vi "prep state ui channel.vi"(7 "instance id":string, 8 "error in":errorcluster, 9 "channel":refnum<class "TBM channel.lvclass">, 10 "ring":refnum<vi>, 11 "engine configuration in":refnum<class "engine configuration.lvclass">) -> (0 "error out":errorcluster, 3 "engine configuration out":refnum<class "engine configuration.lvclass">)   [LabVIEW 2013, in "user tag bus module editor node.lvclass"]
uses:
  user tag bus module editor node.lvclass
  <vilib>/NI/Tag Bus Module Framework/channel/TBM channel.lvclass
  <vilib>/NI/Module Execution Interface/Engine Configuration/engine configuration.lvclass
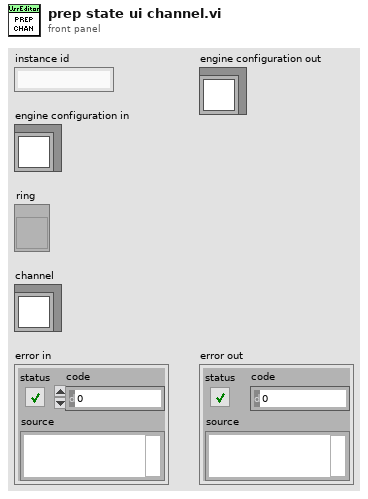
[diagram p1: front panel]
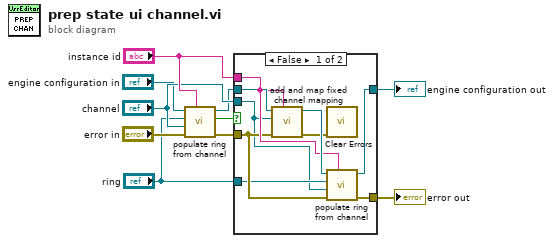
[diagram p0: block diagram]
diagram:
  n1 = call "populate ring from channel.vi"("instance id"="instance id", "error in"="error in", "channel"="channel", "ring"="ring", "engine configuration in"="engine configuration in") -> ("error out"=w8:errorcluster, "mapped"=w4:bool, "engine configuration out"=w6:refnum<class "engine configuration.lvclass">)  [unwired: 4 in]
  n2 = case shown="False" w4 {
    tunnel: [w17 w21] -> w5
    tunnel: w6 -> [w19 w21]
    tunnel: w8 -> [w15 w20]
    tunnel: "channel" -> [w11 _]
    tunnel: "instance id" -> [w16 _]
    tunnel: [w14 w20] -> w9
    tunnel: "ring" -> [w12 _]
    frame False {
      n3 = call <vilib>:"add and map fixed channel mapping.vi"("module instance"=w16, "error in"=w15, "fixed channel"=w11, "engine configuration in"=w19) -> ("error out"=w13:errorcluster, "engine configuration out"=w18:refnum<class "engine configuration.lvclass">)  [unwired: 6 in]
      n4 = call <vilib>:"Clear Errors.vi"("error in (no error)"=w13) -> ()  [unwired: 6 in, 1 out]
      n5 = call "populate ring from channel.vi"("instance id"=w16, "error in"=w15, "channel"=w11, "ring"=w12, "engine configuration in"=w18) -> ("error out"=w14:errorcluster, "engine configuration out"=w17:refnum<class "engine configuration.lvclass">)  [unwired: 4 in, 1 out]
    }
    frame True {
    }
  }
  "error out" <- w9
  "engine configuration out" <- w5
